vi "_Obtain JKISMQ.vi"(8 "Error in":errorcluster caption="Error in (no error)", 9 "create if not found? (T)":bool=TRUE, 11 "Name(\"\" to use uuid) in":string) -> (0 "Error out":errorcluster, 1 "Stand Alone Mode":bool, 3 "JKISMQ":T1, 4 "Name":string)   [LabVIEW 2014, in "JKI-State-Machine-Plus.lvlib"]
uses:
  JKI-State-Machine-Plus.lvlib
  _JKISMQ.ctl
  _Cross JKI StateMachine State Data.ctl
  _Cross JKI StateMachine State Response.ctl
  _JKISMQFGVOPER.ctl
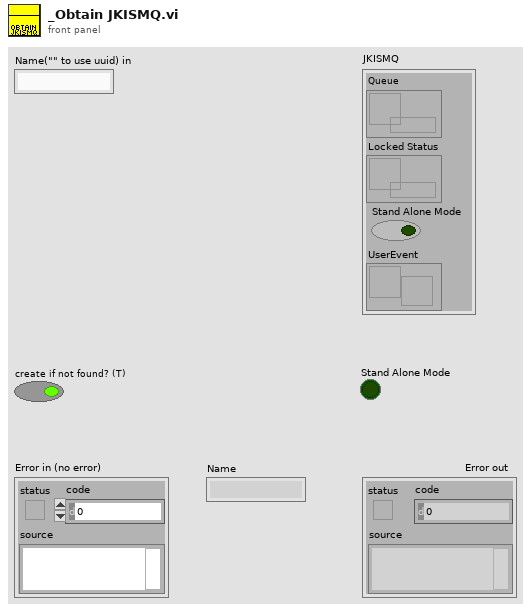
[diagram p1: front panel]
types:
  T1 = typedef "JKI-State-Machine-Plus.lvlib/_JKISMQ.ctl" = cluster{"Queue":refnum<queue>, "Locked Status":refnum<data-value>, "Stand Alone Mode":bool, "UserEvent":refnum<user-event>}
  T2 = typedef "JKI-State-Machine-Plus.lvlib/_JKISMQFGVOPER.ctl" = enum16{"Get By Name", "List", "Check If Name Exists"}
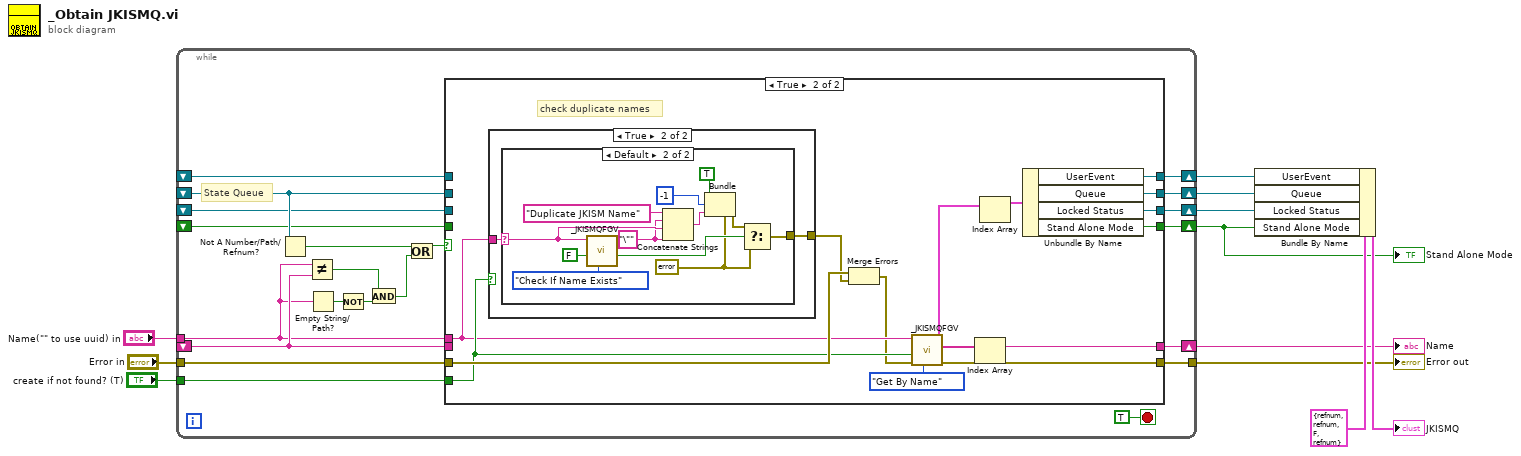
[diagram p0: block diagram]
diagram:
  n1 = while {
    shift-right: [w31] -> w7
    shift-left: _ -> [w29]
    shift-right: [w28] -> w6
    shift-left: _ -> [w20]
    shift-right: [w27] -> w9
    shift-left: _ -> [w26]
    shift-right: [w25] -> w8
    shift-left: _ -> [w24]
    tunnel: "create if not found? (T)" -> [w23]
    tunnel: "Error in" -> [w22]
    tunnel: [w21] -> w3
    tunnel: "Name(\"\" to use uuid) in" -> [w15]
    shift-right: [w13] -> w1
    shift-left: _ -> [w12]
    stop <- TRUE stop-if-true
    # "State Queue"
    n2 = Not A Number/Path/Refnum?(number/path/refnum=w29) -> (NaN/Path/Refnum?=w30:bool)
    n3 = Not Equal?(x=w15, y=w20) -> (x != y?=w18:bool)
    n4 = Empty String/Path?(string/path=w15) -> (empty?=w16:bool)
    n5 = Not(x=w16) -> (.not. x?=w14:bool)
    n6 = And(x=w18, y=w14) -> (x .and. y?=w17:bool)
    n7 = Or(x=w30, y=w17) -> (x .or. y?=w19:bool)
    n8 = case shown="True" w19 {
      tunnel: w20 -> [w37 _]
      tunnel: [w38 w51] -> w31
      tunnel: w29 -> [w38 _]
      tunnel: [w37 w44] -> w28
      tunnel: [w36 w50] -> w27
      tunnel: w26 -> [w36 _]
      tunnel: [w35 w52] -> w25
      tunnel: w24 -> [w35 _]
      tunnel: w23 -> [_ w43]
      tunnel: w22 -> [w34 w47]
      tunnel: [w34 w46] -> w21
      tunnel: w15 -> [_ w42]
      tunnel: [w33 w39] -> w13
      tunnel: w12 -> [w33 _]
      frame False {
      }
      frame True {
        # "check duplicate names"
        n9 = case shown="True" w43 {
          tunnel: w42 -> [_ w54]
          tunnel: [_ w55] -> w40
          frame False {
          }
          frame True {
            n10 = case shown="Default" w54 {
              selector: w54 -> [_ w57]
              tunnel: [_ w64] -> w55
              frame "", "PostMessageAPI", "SendMessageAPI" {
              }
              frame Default {
                w56 = "\"" ("string")
                w63 = errorcluster {"status"=FALSE, "code"=0, "source"=""} ("f")
                n11 = call "_JKISMQFGV.vi"(6:_JKISMQFGVOPER."Check If Name Exists", "create if not found? (T)"=FALSE, "Name(\"\" to use uuid) in"=w57) -> ("Boolean"=w65:bool)  [unwired: 5 in, 3 out]
                n12 = Concatenate Strings("Duplicate JKISM Name" ("String to Prepend to source (\"\")"), w56, w57, w56) -> (w58:string)
                n13 = Bundle(cluster=w63, "status"=TRUE, "code"=-1, "source"=w58) -> (w62:errorcluster)
                n14 = Select(t=w62, s=w65, f=w63) -> (s? t:f=w64:errorcluster)
              }
            }
          }
        }
        n15 = Merge Errors(w47, w40) -> (w41:errorcluster)
        n16 = call "_JKISMQFGV.vi"(6:_JKISMQFGVOPER."Get By Name", "Error in"=w41, "create if not found? (T)"=w43, "Name(\"\" to use uuid) in"=w42) -> ("Error out"=w46:errorcluster, "Name"=w48:string[], "Array"=w53:T1[])  [unwired: 4 in, 1 out]
        n17 = Index Array(array=w48) -> (element=w44:string)  [unwired: 1 in]
        n18 = Index Array(array=w53) -> (element=w45:T1)  [unwired: 1 in]
        n19 = Unbundle By Name(w45) -> ("UserEvent"=w39:refnum<user-event>, "Queue"=w51:refnum<queue>, "Locked Status"=w52:refnum<data-value>, "Stand Alone Mode"=w50:bool)
      }
    }
  }
  "Error out" <- w3
  "Name" <- w6
  "Stand Alone Mode" <- w9
  n20 = Bundle By Name(cluster=T1 {"Queue"=refnum, "Locked Status"=refnum, "Stand Alone Mode"=FALSE, "UserEvent"=refnum} ("JKISMQ"), "UserEvent"=w1, "Queue"=w7, "Locked Status"=w8, "Stand Alone Mode"=w9) -> (→"JKISMQ":T1)
